vi "Destruct.vi"(8 "error in (no error)":errorcluster, 11 "ProjectData in":refnum<class "Project Data.lvclass">) -> (0 "error out":errorcluster)   [LabVIEW 2013, in "SET Project Data.lvlib" / "Project Data.lvclass"]
uses:
  Project Data.lvclass
  Project Data.lvclass/Project Data.ctl
  Resource Data Class/Resource Data.lvclass
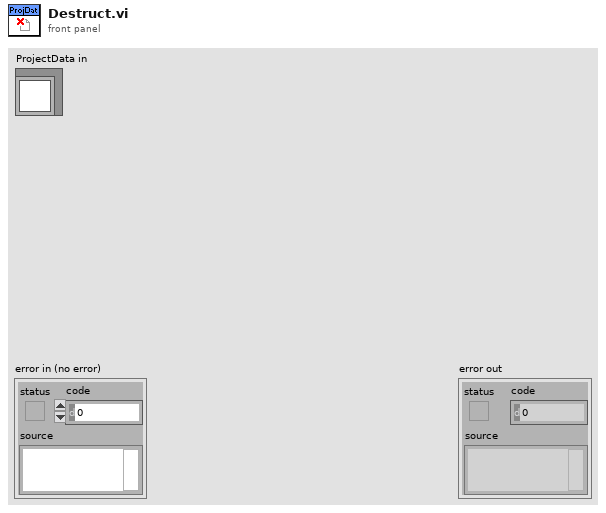
[diagram p1: front panel]
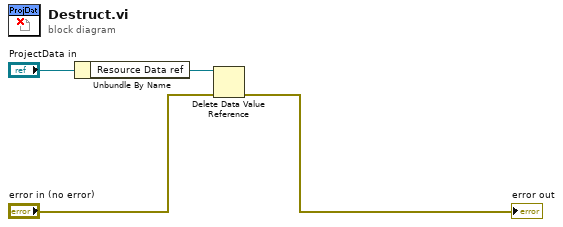
[diagram p0: block diagram]
diagram:
  n1 = Unbundle By Name("ProjectData in") -> ("Resource Data ref"=w3:refnum<data-value>)
  n2 = Delete Data Value Reference(data value reference=w3, error in="error in (no error)") -> (error out=→"error out":errorcluster)  [unwired: 1 out]
